vi "ProcesareNumerica.vi"(11 "image data":T1) -> (1 "image array":dbl[](array[numeric]), 3 "image(28x28)":dbl[][](graph))   [LabVIEW 2024]
uses:
  <vilib>/picture/picture.llb/imagedata.ctl
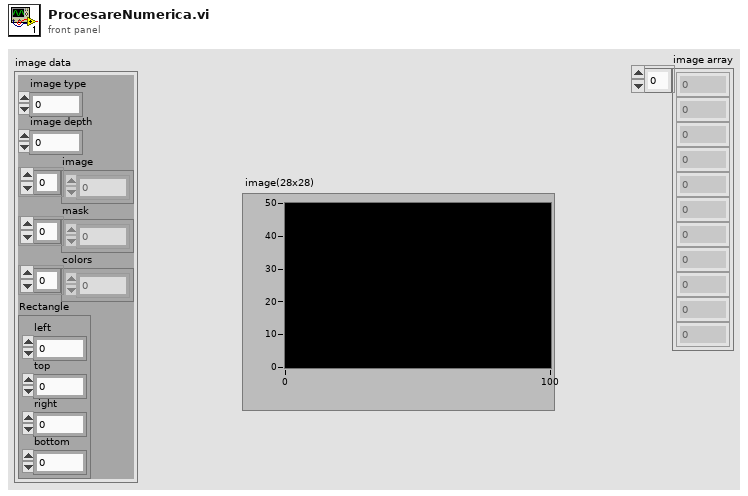
[diagram p1: front panel]
types:
  T1 = typedef "imagedata.ctl" = cluster{"image type":i32, "image depth":i32, "image":u8[], "mask":u8[], "colors":u32[], "Rectangle":cluster{"left":i16, "top":i16, "right":i16, "bottom":i16}}
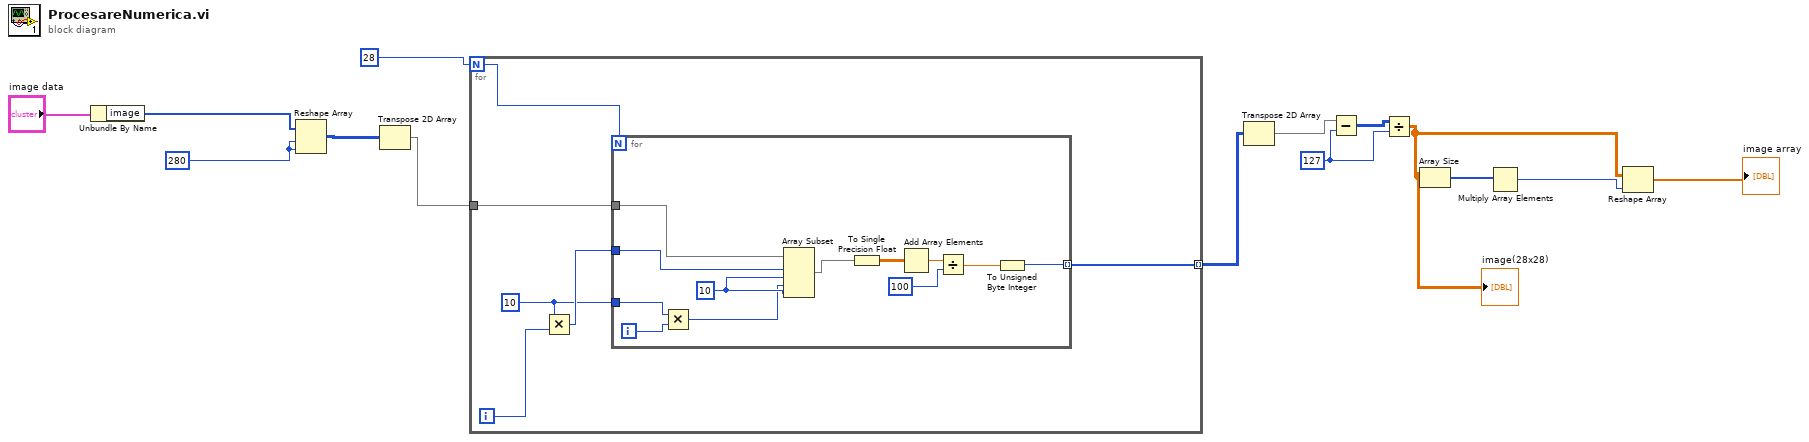
[diagram p0: block diagram]
diagram:
  w6 = 127
  w12 = 280
  n1 = Unbundle By Name("image data") -> ("image"=w13:u8[])
  n2 = Reshape Array(w13, w12, w12) -> (w11:u8[][])
  n3 = Transpose 2D Array(2D array=w11) -> (transposed array=w9:u8[][])
  n4 = for {
    N: 28 -> [w20]
    tunnel: w9 -> [w18]
    tunnel: [w15] -> w8 mode=indexing
    i -> [w19]
    w16 = 10
    n5 = Multiply(x=w16, y=w19) -> (x*y=w17:i32)
    n6 = for {
      N: w20 -> [_]
      tunnel: w18 -> [w32]
      tunnel: w17 -> [w31]
      tunnel: w16 -> [w28]
      tunnel: [w22] -> w15 mode=indexing
      i -> [w29]
      w30 = 10
      n7 = Multiply(x=w28, y=w29) -> (x*y=w27:i32)
      n8 = Array Subset(array=w32, index (row)=w31, length (row)=w30, index (col)=w27, length (col)=w30) -> (w25:u8[][])
      n9 = To Single Precision Float(number=w25) -> (single precision float=w24:sgl[][])
      n10 = Add Array Elements(numeric array=w24) -> (sum=w26:sgl)
      n11 = Divide(x=w26, y=100) -> (x/y=w21:sgl)
      n12 = To Unsigned Byte Integer(number=w21) -> (unsigned 8bit integer=w22:u8)
    }
  }
  n13 = Transpose 2D Array(2D array=w8) -> (transposed array=w7:u8[][])
  n14 = Subtract(x=w7, y=w6) -> (x-y=w5:i32[][])
  n15 = Divide(x=w5, y=w6) -> (x/y=w1:dbl[][])
  "image(28x28)" <- w1
  n16 = Array Size(array=w1) -> (size(s)=w4:i32[])
  n17 = Multiply Array Elements(1:w4) -> (0:w3:i32)
  n18 = Reshape Array "Reshape Array"(w1, w3) -> (→"image array":dbl[])
